vi "Read Formatters.vi"(8 "error in (no error)":errorcluster, 11 "Report Config in":refnum<class "Report Config.lvclass">) -> (0 "error out":errorcluster, 2 "Formatters":refnum<class "Formatter Config.lvclass">[](array[class]), 3 "Report Config out":refnum<class "Report Config.lvclass">)   [LabVIEW 2015, in "Report Config.lvclass"]
uses:
  Report Config.lvclass
  Report Formatters/Base Class/Config/Formatter Config.lvclass
  Report Config.lvclass/Report Config.ctl
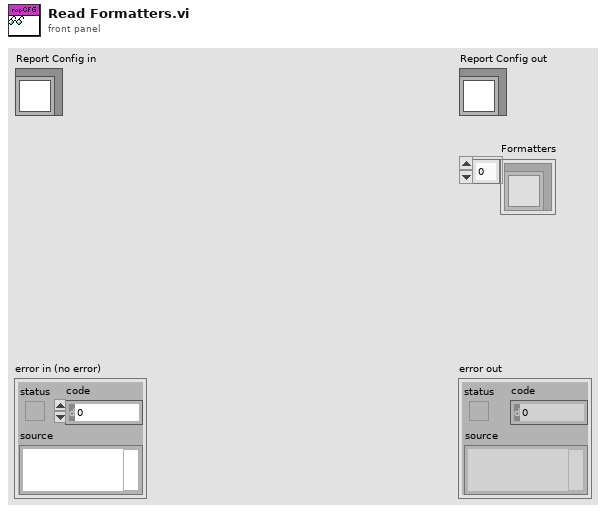
[diagram p1: front panel]
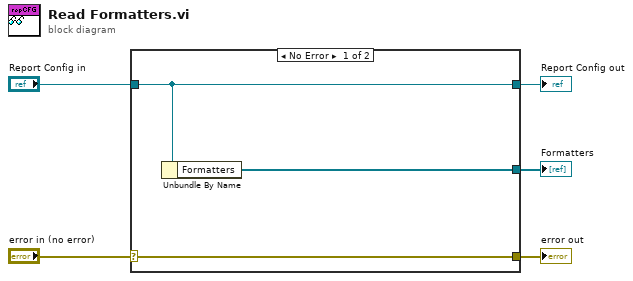
[diagram p0: block diagram]
diagram:
  n1 = case shown="No Error" "error in (no error)" {
    selector: "error in (no error)" -> [w8 w9]
    tunnel: [w8 w9] -> w4
    tunnel: [w7 w10] -> w2
    tunnel: "Report Config in" -> [w7 w10]
    tunnel: [w6 _] -> w1
    frame No Error {
      n2 = Unbundle By Name(w7) -> ("Formatters"=w6:refnum<class "Formatter Config.lvclass">[])
    }
    frame Error {
    }
  }
  "error out" <- w4
  "Report Config out" <- w2
  "Formatters" <- w1
